vi "Create Window.vi"(4 "Height":i32=480, 5 "Title":string, 6 "Width":i32=640, 7 "Flags":u32 format="%.0x", 8 "error in":errorcluster, 10 "Position y":i32, 11 "Position x":i32) -> (0 "error out":errorcluster, 3 "Window Pointer":u32 format="%.0x")   [LabVIEW 2015, in "LibSDL2.lvlib"]
uses:
  LibSDL2.lvlib
  DLL/SDL2.dll
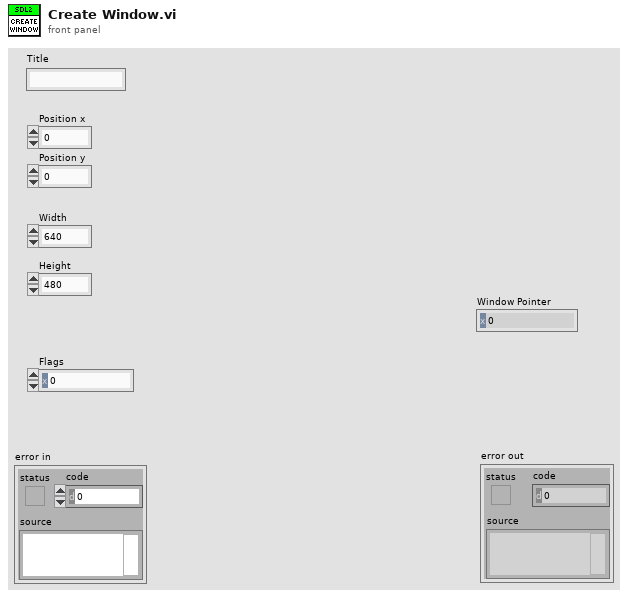
[diagram p1: front panel]
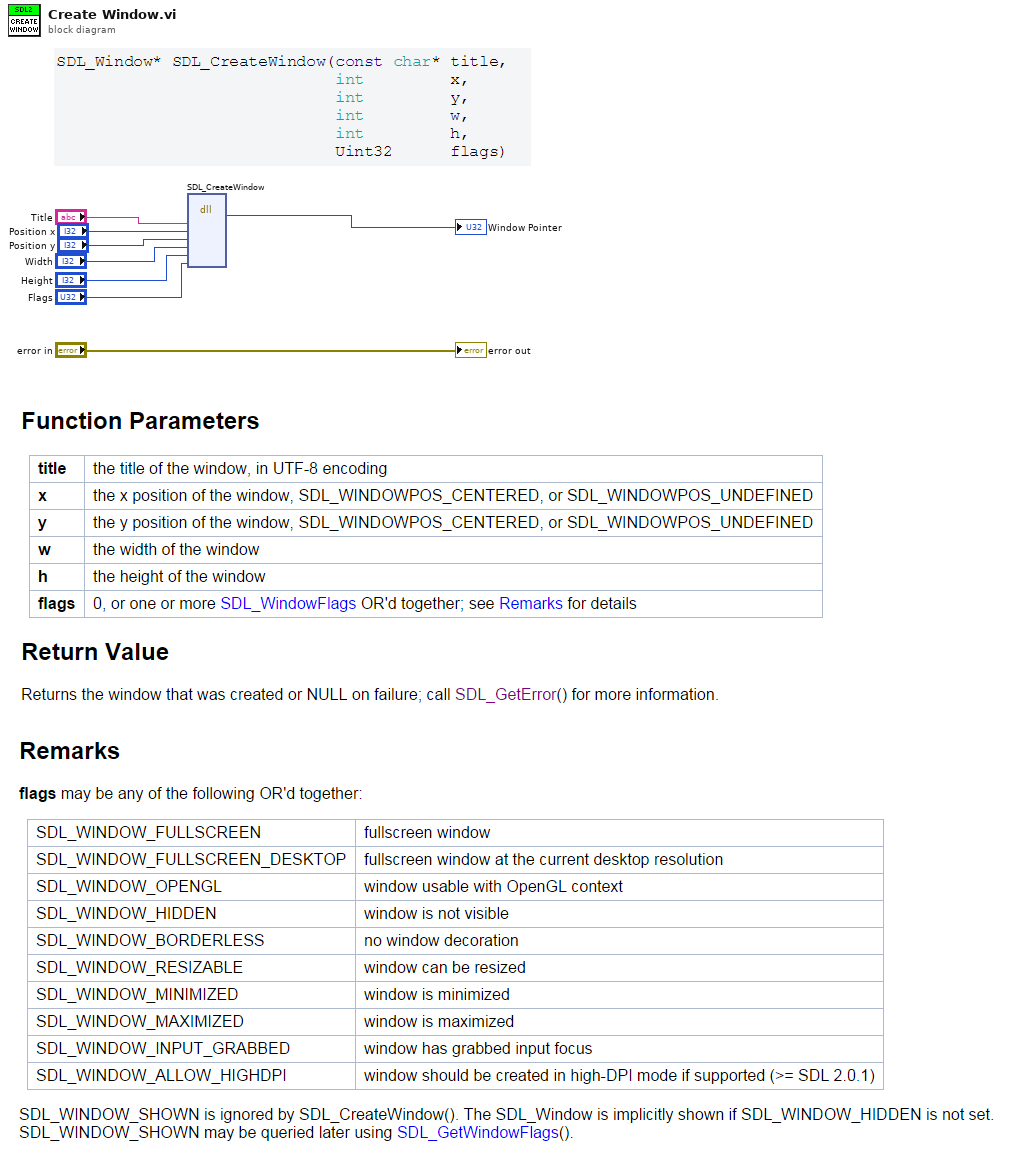
[diagram p0: block diagram]
diagram:
  n1 = dll-call lib="C:/dev/PGS/LabSDL2/Source/Libraries/LibSDL2 Wrapper/DLL/SDL2.dll" fn="SDL_CreateWindow"("title"="Title", "x"="Position x", "y"="Position y", "width"="Width", "height"="Height", "flags"="Flags") -> ("return type"=→"Window Pointer":u32)  [unwired: 9 in, 2 out]
  "error out" <- "error in"
